vi "niDTS WLAN INSTR TX Configure Standards Parameters.vi"(8 "error in (no error)":errorcluster, 11 "niDTS WLAN INSTR TX in":refnum<class "niDTS WLAN INSTR TX.lvclass">) -> (0 "error out":errorcluster, 3 "niDTS WLAN INSTR TX out":refnum<class "niDTS WLAN INSTR TX.lvclass">)   [LabVIEW 2015, in "niDTS WLAN.lvlib" / "niDTS WLAN INSTR TX.lvclass"]
doc: "Sets:\n\n* DataRate\n* McsIndex\n* Nsts\n* FecType\n* GuardInterval"
uses:
  niDTS WLAN INSTR TX.lvclass
  niDTS WLAN INSTR TX.lvclass/niDTS WLAN INSTR TX.ctl
  RiviInstDriver/niRfsaWlan/Objects/niRfsaWlan.lvclass
  niDTS WLAN.lvlib
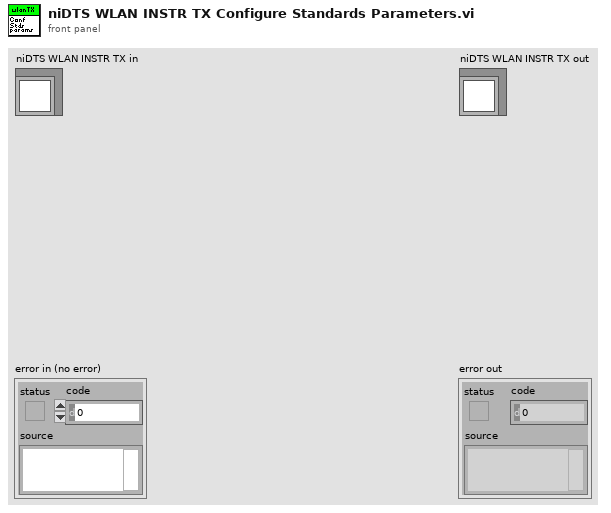
[diagram p1: front panel]
types:
  T1 = enum16{"R1M", "R2M", "R5M5", "R6M", "R9M", "R11M", "R12M", "R18M", "R24M", "R36M", "R48M", "R54M"}
  T2 = enum16{"1M", "2M", "5M5", "6M", "9M", "11M", "12M", "18M", "24M", "36M", "48M", "54M"}
  T3 = typedef "niRfsaWlan.lvclass/niRfsaWlan INC Handle.ctl" = refnum<data-value>
  T4 = typedef "niDTS WLAN.lvlib/niDTS WLAN INC Standard.ctl" = enum16{"802.11 b DSSS", "802.11 a/g OFDM", "802.11 n HT", "802.11 ac VHT"}
  T5 = typedef "niDTS WLAN.lvlib/niDTS WLAN INC DSSS Data Rate.ctl" = enum16{"1", "2", "5.5", "11"}
  T6 = typedef "niDTS WLAN.lvlib/niDTS WLAN INC OFDM Data Rate.ctl" = enum16{"6", "9", "12", "18", "24", "36", "48", "54"}
  T7 = typedef "niDTS WLAN.lvlib/niDTS WLAN INC FEC Coding.ctl" = enum16{"BCC", "LDPC"}
  T8 = typedef "niDTS WLAN.lvlib/niDTS WLAN INC GI.ctl" = enum16{"LONG", "SHORT"}
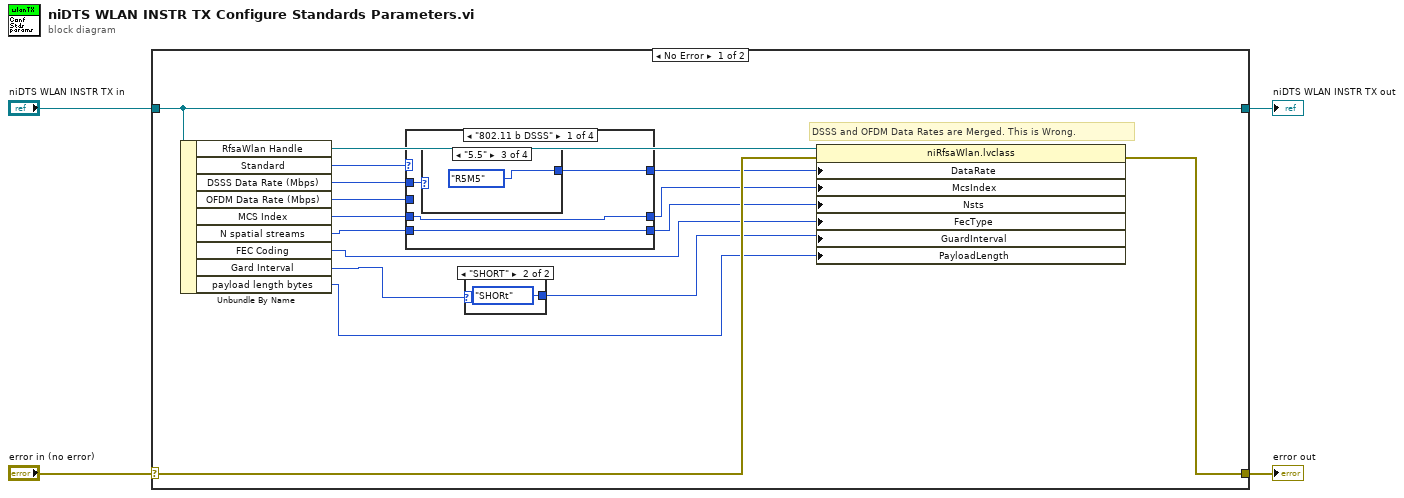
[diagram p0: block diagram]
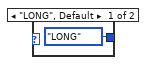
[diagram p2: hidden frame]
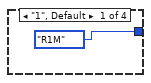
[diagram p3: hidden frame]
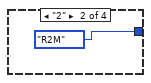
[diagram p4: hidden frame]
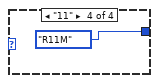
[diagram p5: hidden frame]
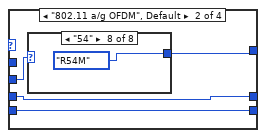
[diagram p6: hidden frame]
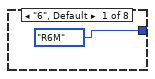
[diagram p7: hidden frame]
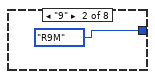
[diagram p8: hidden frame]
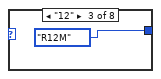
[diagram p9: hidden frame]
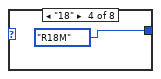
[diagram p10: hidden frame]
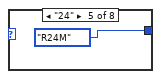
[diagram p11: hidden frame]
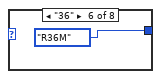
[diagram p12: hidden frame]
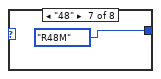
[diagram p13: hidden frame]
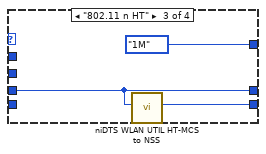
[diagram p14: hidden frame]
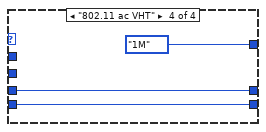
[diagram p15: hidden frame]
diagram:
  n1 = case shown="No Error" "error in (no error)" {
    selector: "error in (no error)" -> [w16 w50]
    tunnel: [w6 w50] -> w3
    tunnel: [w7 w49] -> w1
    tunnel: "niDTS WLAN INSTR TX in" -> [w7 w49]
    frame No Error {
      # "DSSS and OFDM Data Rates are Merged. This is Wrong."
      n2 = Unbundle By Name(w7) -> ("RfsaWlan Handle"=w20:T3, "Standard"=w19:T4, "DSSS Data Rate (Mbps)"=w18:T5, "OFDM Data Rate (Mbps)"=w17:T6, "MCS Index"=w15:i32, "N spatial streams"=w9:i32, "FEC Coding"=w10:T7, "Gard Interval"=w12:T8, "payload length bytes"=w5:i32)
      n3 = case shown="\"802.11 b DSSS\"" w19 {
        tunnel: w18 -> [w26 _ _ _]
        tunnel: w17 -> [_ w34 _ _]
        tunnel: [w25 w33 T2."1M" ("CONFigure:RFSA:WLAN:DataRate") T2."1M" ("CONFigure:RFSA:WLAN:DataRate")] -> w8
        tunnel: w15 -> [w24 w32 w44 w47]
        tunnel: [w24 w32 w44 w47] -> w14
        tunnel: [w23 w31 w43 w46] -> w13
        tunnel: w9 -> [w23 w31 _ w46]
        frame "802.11 b DSSS" {
          n4 = case shown="\"5.5\"" w26 {
            tunnel: [T1."R1M" ("CONFigure:RFSA:WLAN:DataRate") T1."R2M" ("CONFigure:RFSA:WLAN:DataRate") T1."R5M5" ("CONFigure:RFSA:WLAN:DataRate") T1."R11M" ("CONFigure:RFSA:WLAN:DataRate")] -> w25
            frame "1", Default {
            }
            frame "2" {
            }
            frame "5.5" {
            }
            frame "11" {
            }
          }
        }
        frame "802.11 a/g OFDM", Default {
          n5 = case shown="\"54\"" w34 {
            tunnel: [T1."R6M" ("CONFigure:RFSA:WLAN:DataRate") T1."R9M" ("CONFigure:RFSA:WLAN:DataRate") T1."R12M" ("CONFigure:RFSA:WLAN:DataRate") T1."R18M" ("CONFigure:RFSA:WLAN:DataRate") T1."R24M" ("CONFigure:RFSA:WLAN:DataRate") T1."R36M" ("CONFigure:RFSA:WLAN:DataRate") T1."R48M" ("CONFigure:RFSA:WLAN:DataRate") T1."R54M" ("CONFigure:RFSA:WLAN:DataRate")] -> w33
            frame "6", Default {
            }
            frame "9" {
            }
            frame "12" {
            }
            frame "18" {
            }
            frame "24" {
            }
            frame "36" {
            }
            frame "48" {
            }
            frame "54" {
            }
          }
        }
        frame "802.11 n HT" {
          n6 = call "niDTS WLAN UTIL HT-MCS to NSS.vi"("HT MCS"=w44) -> ("NSS"=w43:i32)  [unwired: 10 in]
        }
        frame "802.11 ac VHT" {
        }
      }
      n7 = case shown="\"SHORT\"" w12 {
        tunnel: [enum16{"LONG", "SHORt"}."LONG" ("CONFigure:RFSA:WLAN:MODulation:OFDM:GuardInterval") enum16{"LONG", "SHORt"}."SHORt" ("CONFigure:RFSA:WLAN:MODulation:OFDM:GuardInterval")] -> w11
        frame "LONG", Default {
        }
        frame "SHORT" {
        }
      }
      n8 = property class="niRfsaWlan.lvclass"(reference=w20, error in=w16, "DataRate"=w8, "McsIndex"=w14, "Nsts"=w13, "FecType"=w10, "GuardInterval"=w11, "PayloadLength"=w5) -> (error out=w6:errorcluster)  [unwired: 1 out]
    }
    frame Error {
    }
  }
  "error out" <- w3
  "niDTS WLAN INSTR TX out" <- w1
